vi "GV ScanGalvoDelay_tick.vi"() -> ()   [LabVIEW 2017]
panel:
  in  "ScanGalvoDelay_tick":u32
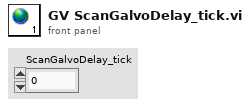
[diagram p1: front panel]
diagram:
